vi "wrap.PushBool.vi"(0 "class.GLue in":refnum<class "class.GLue.lvclass">, 7 "Boolean":bool, 11 "error in (no error)":errorcluster) -> (4 "class.GLue out":refnum<class "class.GLue.lvclass">, 15 "error out":errorcluster)   [LabVIEW 2014, in "GLue.lvlib" / "class.GLue.lvclass"]
uses:
  class.GLue.lvclass
  class.GLue.lvclass/class.GLue.ctl
  Resources/GLue.dll
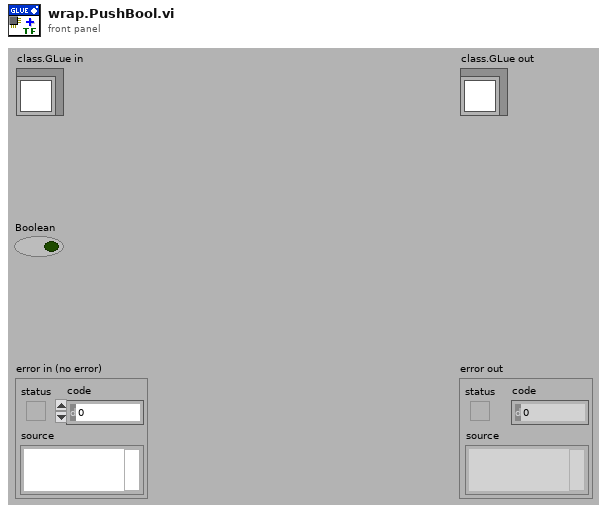
[diagram p1: front panel]
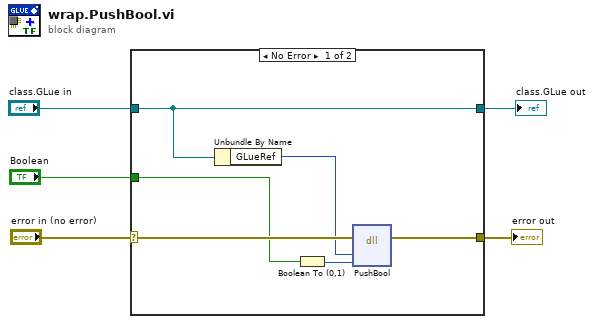
[diagram p0: block diagram]
diagram:
  n1 = case shown="No Error" "error in (no error)" {
    selector: "error in (no error)" -> [w10 w13]
    tunnel: [w9 w13] -> w4
    tunnel: [w11 w12] -> w2
    tunnel: "class.GLue in" -> [w11 w12]
    tunnel: "Boolean" -> [w6 _]
    frame No Error {
      n2 = Unbundle By Name(w11) -> ("GLueRef"=w8:i64)
      n3 = Boolean To (0,1)(Boolean=w6) -> (0, 1=w7:i16)
      n4 = dll-call lib="C:/Users/Antonie/Documents/work/glue/trunk/Resources/GLue.dll" fn="PushBool"(error in=w10, "MLua"=w8, "Bool"=w7) -> (error out=w9:errorcluster)  [unwired: 5 in, 1 out]
    }
    frame Error {
    }
  }
  "error out" <- w4
  "class.GLue out" <- w2
